vi "Pixel Counter (SubVI).vi"(5 "Image Height":u16=65535, 7 "Image Width":u16=65535, 8 "Pixel Valid":bool) -> (3 "Pixel Bus":T1)   [LabVIEW 2015]
uses:
  Pixel Bus.ctl
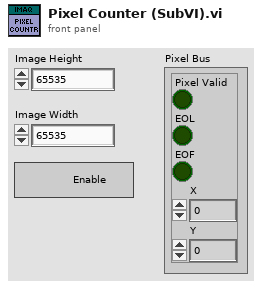
[diagram p1: front panel]
types:
  T1 = typedef "Pixel Bus.ctl" = cluster{"Pixel Valid":bool, "EOL":bool, "EOF":bool, "X":u16, "Y":u16}
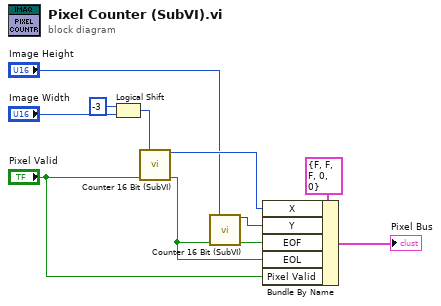
[diagram p0: block diagram]
diagram:
  n1 = Logical Shift(y=i16 -3, x="Image Width") -> (x << y=w11:u16)
  n2 = call "Counter 16 Bit (SubVI).vi"("Max. Count"=w11, "Enable"="Pixel Valid") -> ("Count"=w8:u16, "Count End?"=w4:bool)  [unwired: 11 in, 1 out]
  n3 = call "Counter 16 Bit (SubVI).vi"("Max. Count"="Image Height", "Enable"=w4) -> ("Count"=w7:u16, "Count End?"=w6:bool)  [unwired: 11 in, 1 out]
  n4 = Bundle By Name(cluster=T1 {"Pixel Valid"=FALSE, "EOL"=FALSE, "EOF"=FALSE, "X"=0, "Y"=0}, "X"=w8, "Y"=w7, "EOF"=w6, "EOL"=w4, "Pixel Valid"="Pixel Valid") -> (→"Pixel Bus":T1)
